vi "Compute Checksum.vi"(11 "Command":u8[](array[numeric])) -> (3 "Checksum":u16)   [LabVIEW 2010]
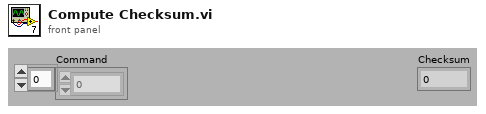
[diagram p1: front panel]
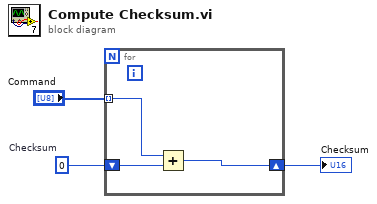
[diagram p0: block diagram]
diagram:
  w2 = u16 0  # Checksum
  n1 = for {
    shift-right: [w5] -> w1
    shift-left: w2 -> [w6]
    tunnel: "Command" -> [w4] mode=indexing
    n2 = Add(x=w4, y=w6) -> (x+y=w5:u16)
  }
  "Checksum" <- w1
